vi "MoveMultiDrives.vi"(0 "Start Counter":dbl[](array[numeric]), 1 "Channel Properties":T1[](array[typedef]) {"Current Pos" format="%.2f"; "Backlash/Eng units" format="%.2f"; "Pulses/rev" format="%.2f"; "Pos Tolerance" format="%.2f"; "Pulses/unit" format="%.2f"; "Acc. Min" format="%.2f"; "Acc. Max" format="%.2f"; "Vel. Min" format="%.2f"; "Vel. Max" format="%.2f"; "Acc. Default" format="%.2f"; "Vel. Default" format="%.2f"}, 2 "GoTo Array (pulse position, some channels)":T4[](array[typedef]) {"Acceleration" format="%.2f"; "Velocity" format="%.2f"; "Go To Position" step=100000.0}, 3 "Final move":bool, 4 "Predicted Move Time":dbl format="%.2f") -> (5 "Error string":string, 6 "Stop Pressed?":bool, 7 "Channel Properties Out":T1[](array[typedef]) {"Current Pos" format="%.2f"; "Backlash/Eng units" format="%.2f"; "Pulses/rev" format="%.2f"; "Pos Tolerance" format="%.2f"; "Pulses/unit" format="%.2f"; "Acc. Min" format="%.2f"; "Acc. Max" format="%.2f"; "Vel. Min" format="%.2f"; "Vel. Max" format="%.2f"; "Acc. Default" format="%.2f"; "Vel. Default" format="%.2f"})   [LabVIEW 2022 SP3]
uses:
  ~subVIs/DriveClusterLower.ctl
  ~subVIs/DriveStatus.ctl
  ~subVIs/DriveProperties.ctl
  ~subVIs/Traverse Type.ctl
  ~subVIs/GenericDriveCommand.ctl
  Dynamixel/Sub Vis/Dynamixel Commands.ctl
  ~subVIs/DriveConfigGlobal.vi
  Anemometry/Anemometry Sub Vis/Globals/Trav_pos_global.vi
panel:
  out "Actual Travel Time":dbl format="%#.3g"
  out "Case":string
  out "Working?":bool
  out "ErrorMagnitude":dbl
  out "Move On Track?":bool
  out "Log File":path
  out "Move Terminated on Timeout":bool
  in  "Axis info cluster":T3
  out "Start Time":dbl format="%.2f"
  out "Bar2":dbl(slide)=2.0 scale=-23355.245670318604..-23317.840270996094
  out "Bar1":dbl(slide)=2.0 scale=-142950.39999389648..-143360.0
  out "Bar0":dbl(slide)=2.0 scale=228853.125..229365.0
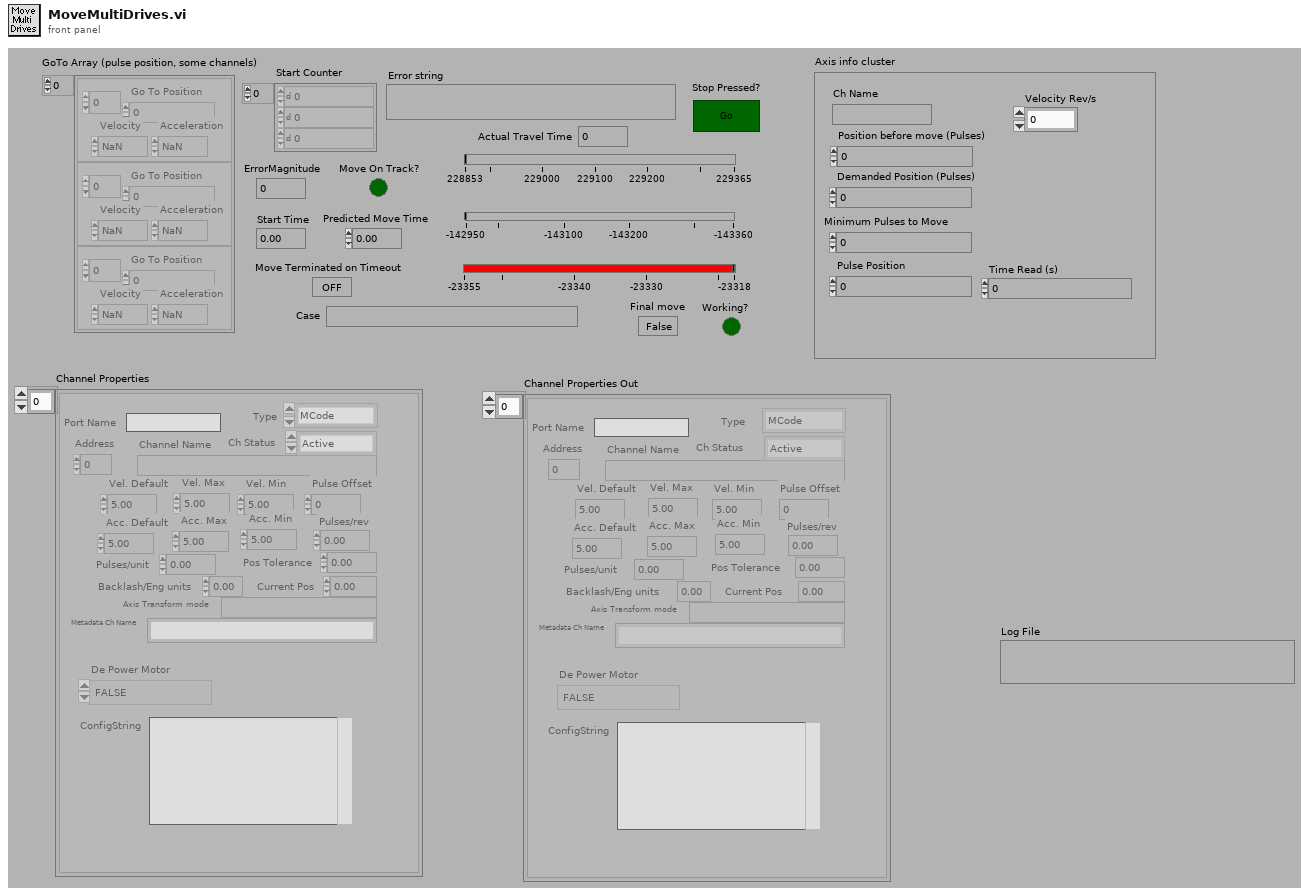
[diagram p1: front panel]
types:
  T1 = typedef "DriveProperties.ctl" = cluster{"Channel Name":string, "Vel. Default":sgl, "Acc. Default":sgl, "Vel. Max":sgl, "Vel. Min":sgl, "Acc. Max":sgl, "Acc. Min":sgl, "Pulses/unit":sgl, "Address":u8, "Pulse Offset":i32, "Pos Tolerance":sgl, "Pulses/rev":sgl, "Backlash/Eng units":sgl, "Current Pos":sgl, "Ch Status":enum16{"Active", "Offline", "Simulate"}, "Port Name":string, "Axis Transform mode":string, "Metadata Ch Name":string, "Type":T2, "De Power Motor":enum16{"TRUE", "FALSE"}, "ConfigString":string}
  T2 = typedef "Traverse Type.ctl" = enum16{"MCode", "Dynamixel"}
  T3 = typedef "DriveStatus.ctl" = cluster{"Ch Name":string, "Position before move (Pulses)":dbl, "Demanded Position (Pulses)":dbl, "Minimum Pulses to Move":dbl, "Pulse Position":dbl, "Time Read (s)":dbl, "Velocity Rev/s":dbl}
  T4 = typedef "DriveClusterLower.ctl" = cluster{"Go To Position":dbl, "Velocity":dbl, "Acceleration":dbl, "Address":u8}
  T5 = typedef "GenericDriveCommand.ctl" = string
  T6 = typedef "Dynamixel Commands.ctl" = enum16{"Torque Enable", "Present Position", "Threshold", "Max Position Limit", "Acceleration Profile", "Velocity Profile", "Goal Position", "Position Proportional Gain", "Position Integral Gain", "Position Differential Gain ", "Shutdown", "Write Operating Mode", "Read Operating Mode"}
  T7 = cluster{"GenericDriveCommand":T5, "Go To Position":dbl}
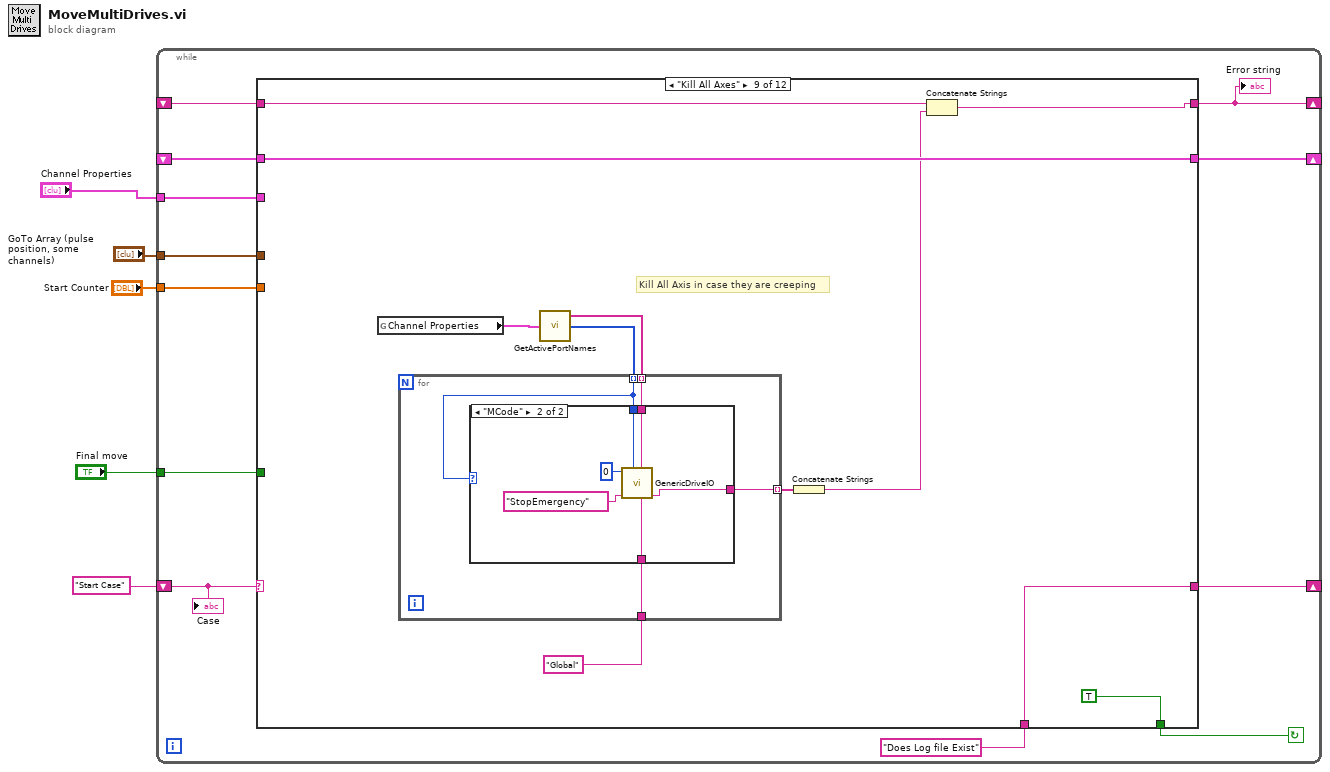
[diagram p0: block diagram]
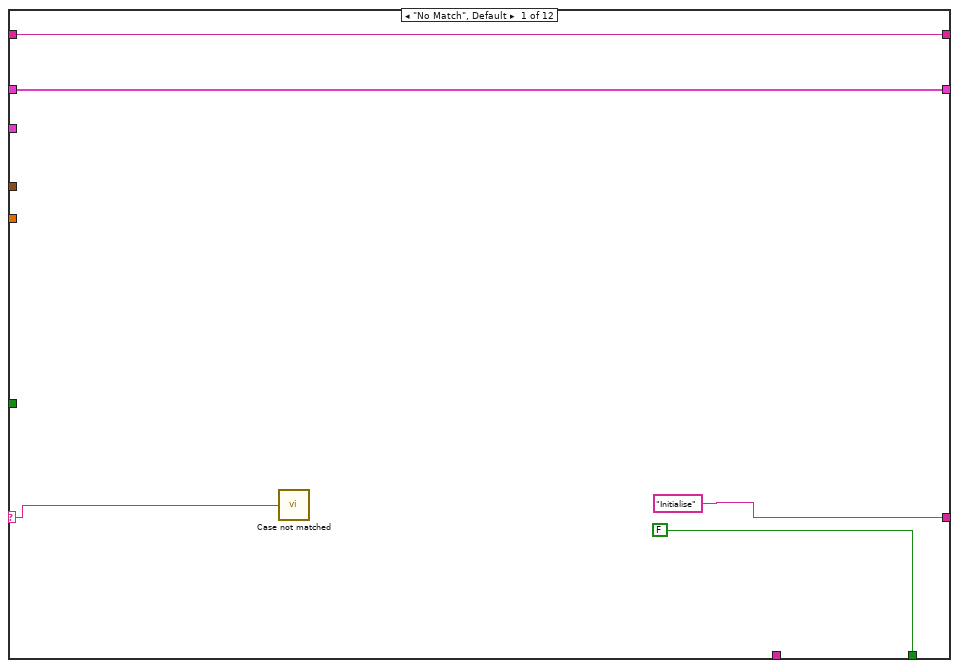
[diagram p2: hidden frame]
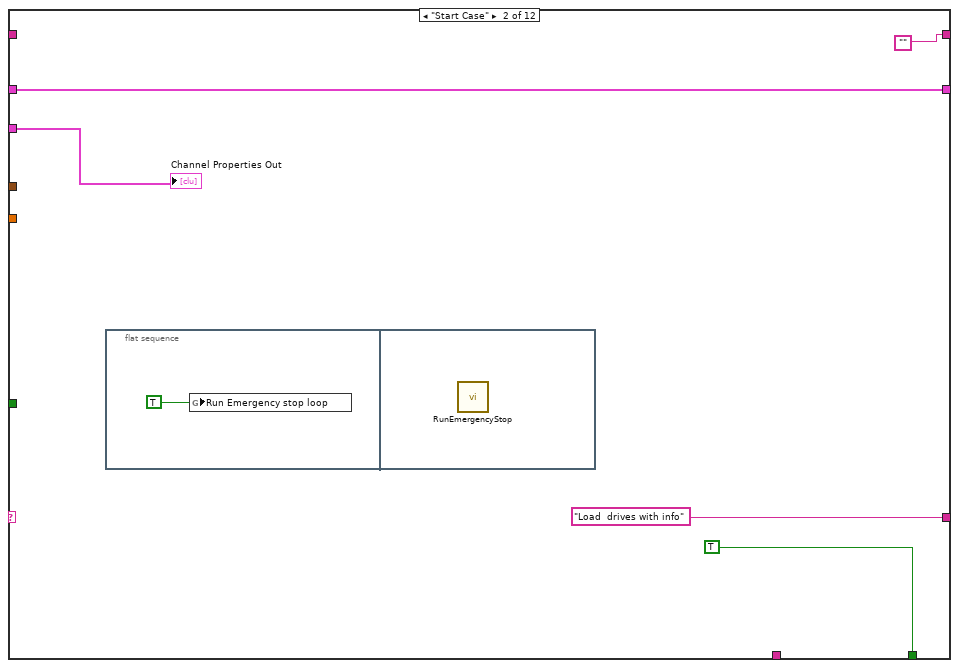
[diagram p3: hidden frame]
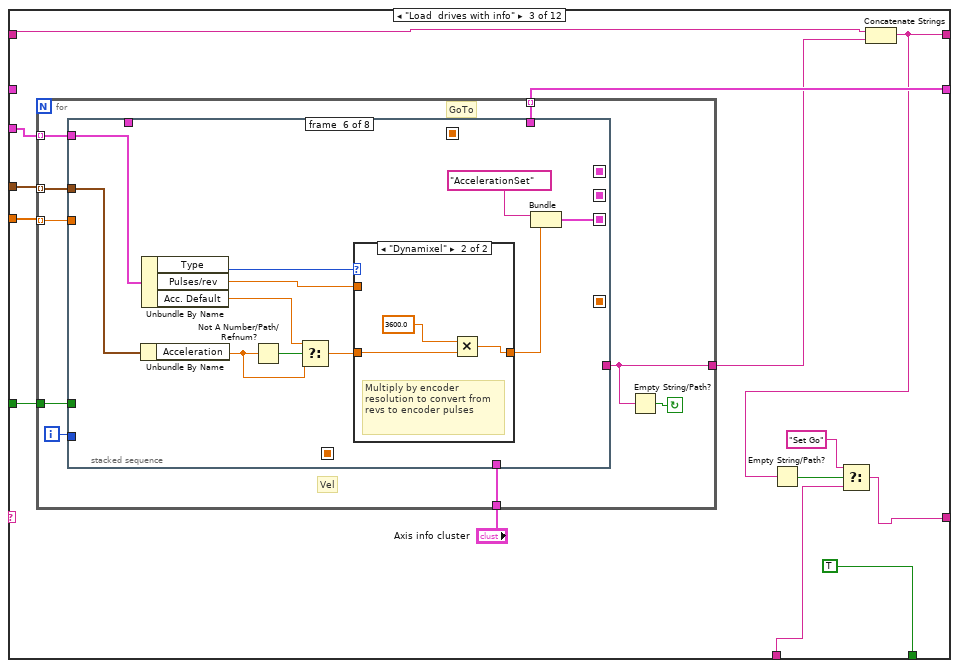
[diagram p4: hidden frame]
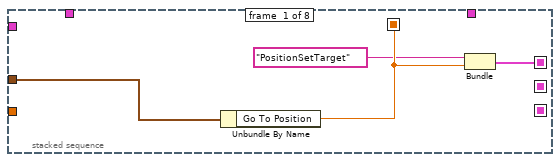
[diagram p5: hidden frame]
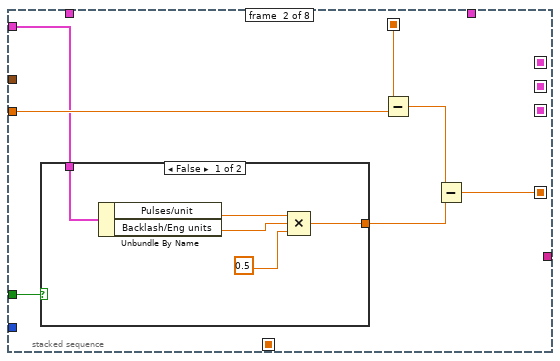
[diagram p6: hidden frame]
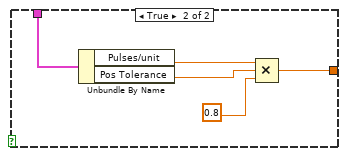
[diagram p7: hidden frame]
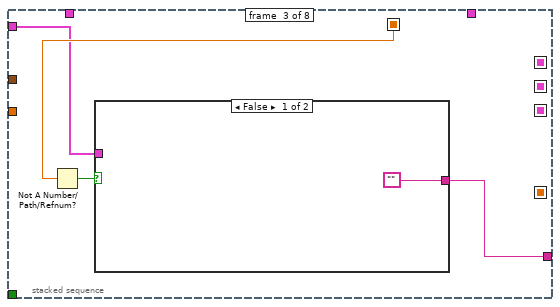
[diagram p8: hidden frame]
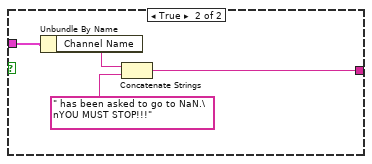
[diagram p9: hidden frame]
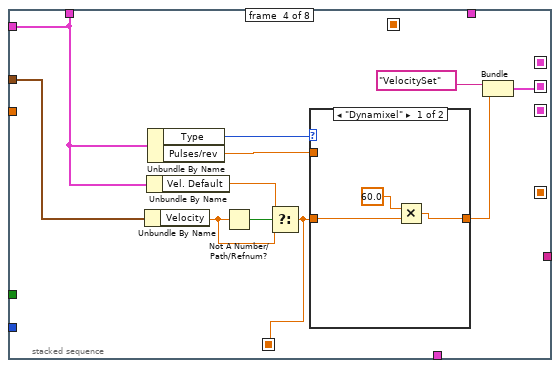
[diagram p10: hidden frame]
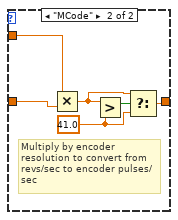
[diagram p11: hidden frame]
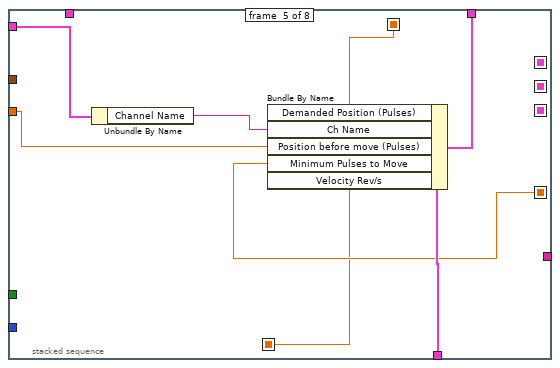
[diagram p12: hidden frame]
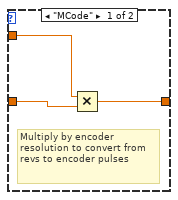
[diagram p13: hidden frame]
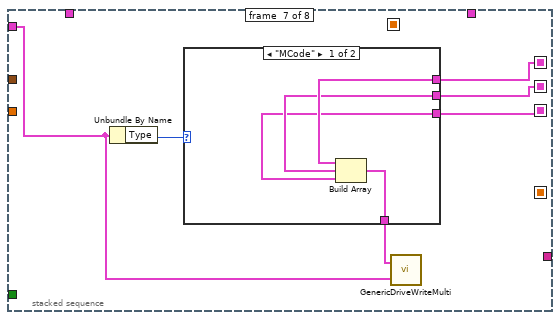
[diagram p14: hidden frame]
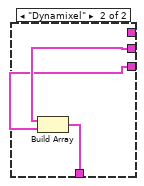
[diagram p15: hidden frame]
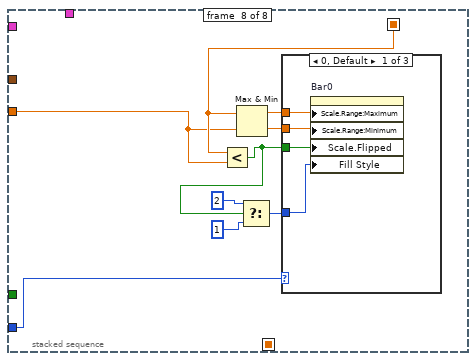
[diagram p16: hidden frame]
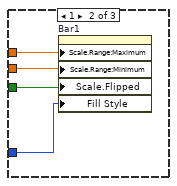
[diagram p17: hidden frame]
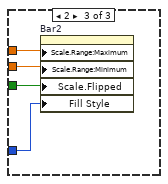
[diagram p18: hidden frame]
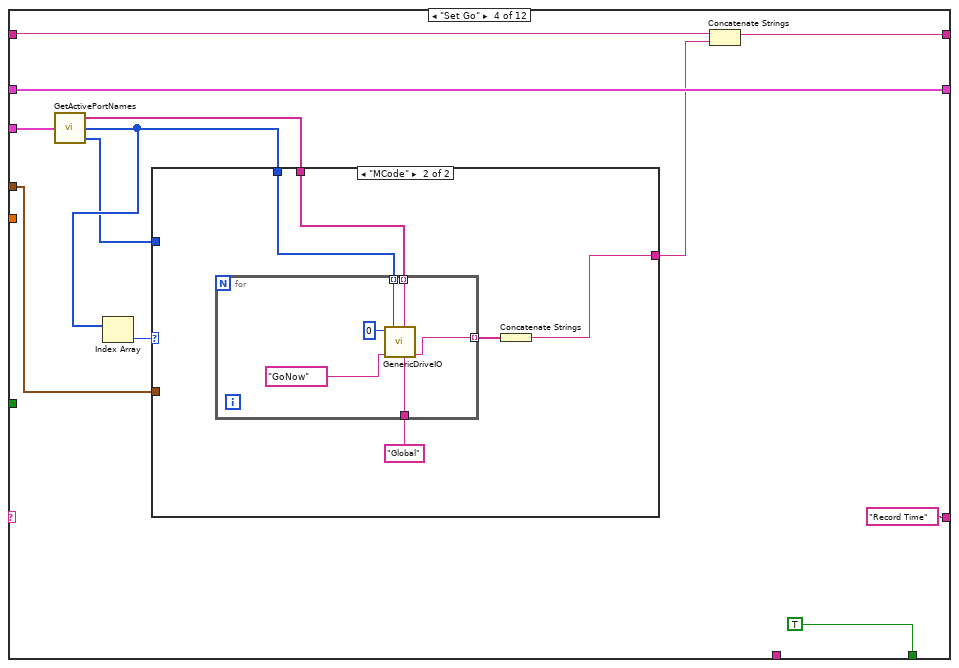
[diagram p19: hidden frame]
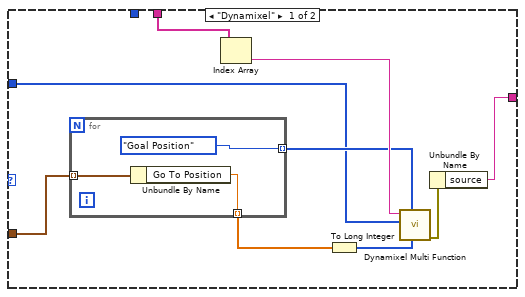
[diagram p20: hidden frame]
diagram:
  n1 = while {
    shift-left: _ -> [w12]
    shift-right: [w11] -> _
    tunnel: "Final move" -> [w13]
    tunnel: "Start Counter" -> [w14]
    tunnel: "GoTo Array (pulse position, some channels)" -> [w15]
    tunnel: "Channel Properties" -> [w16]
    shift-left: "Start Case" -> [w17]
    shift-right: [w7] -> _
    shift-right: [w6] -> _
    shift-left: _ -> [w10]
    stop <- w9 continue-if-true
    n2 = case shown="\"Kill All Axes\"" w17 {
      selector: w17 -> [w19 _ _ _ _ _ _ _ _ _ _ _]
      tunnel: [FALSE TRUE TRUE TRUE TRUE TRUE TRUE TRUE TRUE TRUE TRUE FALSE] -> w9
      tunnel: ["Initialise" "Load  drives with info" w30 "Record Time" "Check status of axis" w209 "Continue looping?" w359 w391 w419 "Write to Log file" "End"] -> w7
      tunnel: w16 -> [_ w23 w29 w162 _ w204 w253 w355 _ _ _ _]
      tunnel: w15 -> [_ _ w41 w163 _ _ w261 w353 _ _ _ _]
      tunnel: w14 -> [_ _ w40 _ _ _ w260 _ _ _ _ _]
      tunnel: w13 -> [_ _ w39 _ _ _ _ _ _ _ _ _]
      tunnel: [w20 w25 w37 w170 w199 w218 w259 w362 w395 w414 w441 w463] -> w11
      tunnel: w12 -> [w20 w25 _ w170 w199 w203 w259 w362 w395 w414 w441 w463]
      tunnel: w10 -> [w18 _ w36 w168 w197 w207 w256 w338 w389 w415 w423 w462]
      tunnel: [w18 "" w34 w167 w197 w205 w254 w338 w387 w415 w423 w462] -> w6
      tunnel: "Does Log file Exist" -> [_ _ w31 _ _ _ _ _ w391 _ _ _]
      frame "No Match", Default {
        n3 = call "Case not matched.vi"("Case Name not Matched"=w19) -> ()
      }
      frame "Start Case" {
        n4 = flat-sequence {
          frame #0 {
            n5 = global write "DriveConfigGlobal.vi" "Run Emergency stop loop"(TRUE) -> ()
          }
          frame #1 {
            n6 = call "RunEmergencyStop.vi"() -> ()  [unwired: 1 in, 7 out]
          }
        }
        "Channel Properties Out" <- w23
      }
      frame "Load  drives with info" {
        n7 = for {
          tunnel: w41 -> [w50] mode=indexing
          tunnel: w40 -> [w49] mode=indexing
          tunnel: w39 -> [w48]
          tunnel: "Axis info cluster" -> [w47]
          tunnel: [w46] -> w37 mode=indexing
          tunnel: [w45] -> w35
          tunnel: w29 -> [w43] mode=indexing
          i -> [w51]
          stop <- w44 continue-if-true
          # "Vel"
          # "GoTo"
          n8 = stacked-sequence {
            seq-local: [w54 _ _ _ _ _ _ _] -> [_ w62 w76 _ w104 _ _ w145]
            seq-local: [w53 _ _ _ _ _ _ _] -> [_ _ _ _ _ _ w132 _]
            seq-local: [_ _ _ w88 _ _ _ _] -> [_ _ _ _ _ _ w131 _]
            seq-local: [_ _ _ _ _ w117 _ _] -> [_ _ _ _ _ _ w130 _]
            seq-local: [_ w58 _ _ _ _ _ _] -> [_ _ _ _ w108 _ _ _]
            seq-local: [_ _ _ w83 _ _ _ _] -> [_ _ _ _ w103 _ _ _]
            tunnel: w50 -> [w55 _ _ w92 _ w120 _ _]
            tunnel: w51 -> [_ _ _ _ _ _ _ w146]
            tunnel: w48 -> [_ w60 _ _ _ _ _ _]
            tunnel: [_ _ _ w82 _ _ _ _] -> _
            tunnel: w49 -> [_ w59 _ _ w106 _ _ w144]
            tunnel: w47 -> [_ _ _ _ w109 _ _ _]
            tunnel: [_ _ _ _ w107 _ _ _] -> w46
            tunnel: [_ _ w74 _ _ _ _ _] -> w45
            tunnel: w43 -> [_ w56 w73 w82 w102 w112 w127 _]
            frame #0 {
              n9 = Unbundle By Name(w55) -> ("Go To Position"=w54:dbl)
              n10 = Bundle("GenericDriveCommand"=T5 "PositionSetTarget", "Go To Position"=w54) -> (w53:T7)  [unwired: 1 out]
            }
            frame #1 {
              n11 = case shown="False" w60 {
                tunnel: w56 -> [w67 w72]
                tunnel: [w63 w68] -> w61
                frame False {
                  n12 = Unbundle By Name(w67) -> ("Pulses/unit"=w66:sgl, "Backlash/Eng units"=w65:sgl)
                  n13 = Compound Arithmetic op=MULTIPLY(w66, w65, 0.5) -> (w63:dbl)
                }
                frame True {
                  n14 = Unbundle By Name(w72) -> ("Pulses/unit"=w71:sgl, "Pos Tolerance"=w70:sgl)
                  n15 = Compound Arithmetic op=MULTIPLY(w71, w70, 0.8) -> (w68:dbl)
                }
              }
              n16 = Subtract(x=w62, y=w59) -> (x-y=w57:dbl)
              n17 = Subtract(x=w57, y=w61) -> (x-y=w58:dbl)
            }
            frame #2 {
              n18 = Not A Number/Path/Refnum?(number/path/refnum=w76) -> (NaN/Path/Refnum?=w75:bool)
              n19 = case shown="False" w75 {
                tunnel: w73 -> [_ w81]
                tunnel: ["" w80] -> w74
                frame False {
                }
                frame True {
                  n20 = Unbundle By Name(w81) -> ("Channel Name"=w79:string)
                  n21 = Concatenate Strings(w79, " has been asked to go to NaN.\nYOU MUST STOP!!!") -> (w80:string)
                }
              }
            }
            frame #3 {
              n22 = Unbundle By Name(w92) -> ("Velocity"=w89:dbl)
              n23 = Unbundle By Name(w82) -> ("Vel. Default"=w90:sgl)
              n24 = Unbundle By Name(w82) -> ("Type"=w86:T2, "Pulses/rev"=w85:sgl)
              n25 = Not A Number/Path/Refnum?(number/path/refnum=w89) -> (NaN/Path/Refnum?=w91:bool)
              n26 = Select(t=w90, s=w91, f=w89) -> (s? t:f=w83:dbl)
              n27 = case shown="\"Dynamixel\"" w86 {
                tunnel: w83 -> [w95 w96]
                tunnel: w85 -> [_ w101]
                tunnel: [w93 w100] -> w84
                frame "Dynamixel" {
                  n28 = Multiply(x=60.0, y=w95) -> (x*y=w93:dbl)
                }
                frame "MCode" {
                  w97 = 41.0 ("y")
                  # "Multiply by encoder resolution to convert from revs/sec to encoder pulses/sec"
                  n29 = Multiply(x=w101, y=w96) -> (x*y=w98:dbl)
                  n30 = Greater?(x=w98, y=w97) -> (0:w99:bool)
                  n31 = Select(t=w98, s=w99, f=w97) -> (s? t:f=w100:dbl)
                }
              }
              n32 = Bundle("GenericDriveCommand"=T5 "VelocitySet", "y"=w84) -> (w88:cluster{"GenericDriveCommand":T5, "y":dbl})  [unwired: 1 out]
            }
            frame #4 {
              n33 = Unbundle By Name(w102) -> ("Channel Name"=w105:string)
              n34 = Bundle By Name(cluster=w109, "Demanded Position (Pulses)"=w104, "Ch Name"=w105, "Position before move (Pulses)"=w106, "Minimum Pulses to Move"=w108, "Velocity Rev/s"=w103) -> (w107:T3)
            }
            frame #5 {
              n35 = Unbundle By Name(w120) -> ("Acceleration"=w118:dbl)
              n36 = Unbundle By Name(w112) -> ("Type"=w111:T2, "Pulses/rev"=w115:sgl, "Acc. Default"=w110:sgl)
              n37 = Not A Number/Path/Refnum?(number/path/refnum=w118) -> (NaN/Path/Refnum?=w119:bool)
              n38 = Select(t=w110, s=w119, f=w118) -> (s? t:f=w114:dbl)
              n39 = case shown="\"Dynamixel\"" w111 {
                tunnel: w114 -> [w123 w126]
                tunnel: w115 -> [w121 _]
                tunnel: [w122 w124] -> w113
                frame "MCode" {
                  # "Multiply by encoder resolution to convert from revs to encoder pulses"
                  n40 = Multiply(x=w121, y=w123) -> (x*y=w122:dbl)
                }
                frame "Dynamixel" {
                  # "Multiply by encoder resolution to convert from revs to encoder pulses"
                  n41 = Multiply(x=3600.0, y=w126) -> (x*y=w124:dbl)
                }
              }
              n42 = Bundle("GenericDriveCommand"=T5 "AccelerationSet", w113) -> (w117:cluster{"GenericDriveCommand":T5, dbl})  [unwired: 1 out]
            }
            frame #6 {
              n43 = Unbundle By Name(w127) -> ("Type"=w128:T2)
              n44 = case shown="\"MCode\"" w128 {
                tunnel: w132 -> [w136 _]
                tunnel: w131 -> [w135 w139]
                tunnel: w130 -> [w134 w138]
                tunnel: [w133 w137] -> w129
                frame "MCode" {
                  n45 = Build Array(w136, w135, w134) -> (w133:cluster{"GenericDriveCommand":T5, "y":dbl}[])
                }
                frame "Dynamixel" {
                  n46 = Build Array(w139, w138) -> (w137:cluster{"GenericDriveCommand":T5, "y":dbl}[])
                }
              }
              n47 = call "GenericDriveWriteMulti.vi"("Channel Description"=w127, "Array Constant"=w129) -> ()  [unwired: 4 in, 1 out]
            }
            frame #7 {
              n48 = Less?(x=w145, y=w144) -> (x < y?=w143:bool)
              n49 = Max & Min(x=w145, y=w144) -> (max(x,y)=w148:dbl, min(x,y)=w147:dbl)
              n50 = Select(t=2, s=w143, f=1 ("Fill Style")) -> (s? t:f=w140:i32)
              n51 = case shown="0, Default" w146 {
                tunnel: w148 -> [w152 w156 w160]
                tunnel: w147 -> [w151 w155 w159]
                tunnel: w143 -> [w150 w154 w158]
                tunnel: w140 -> [w149 w153 w157]
                frame 0, Default {
                  n52 = property on="Bar0" class="Slide (strict)"("Scale.Range:Maximum"=w152, "Scale.Range:Minimum"=w151, "Scale.Flipped"=w150, "Fill Style"=w149) -> ()  [unwired: 2 in, 2 out]
                }
                frame 1 {
                  n53 = property on="Bar1" class="Slide (strict)"("Scale.Range:Maximum"=w156, "Scale.Range:Minimum"=w155, "Scale.Flipped"=w154, "Fill Style"=w153) -> ()  [unwired: 2 in, 2 out]
                }
                frame 2 {
                  n54 = property on="Bar2" class="Slide (strict)"("Scale.Range:Maximum"=w160, "Scale.Range:Minimum"=w159, "Scale.Flipped"=w158, "Fill Style"=w157) -> ()  [unwired: 2 in, 2 out]
                }
              }
            }
          }
          n55 = Empty String/Path?(string/path=w45) -> (empty?=w44:bool)
        }
        n56 = Concatenate Strings(w36, w35) -> (w34:string)
        n57 = Empty String/Path?(string/path=w34) -> (empty?=w33:bool)
        n58 = Select(t="Set Go", s=w33, f=w31) -> (s? t:f=w30:string)
      }
      frame "Set Go" {
        n59 = call "GetActivePortNames.vi"("Channel Properties"=w162) -> ("Port Name Array"=w169:string[], "Drive Type Array"=w165:T2[], "Address"=w161:u8[])
        n60 = Index Array(array=w165) -> (element=w164:T2)  [unwired: 1 in]
        n61 = case shown="\"MCode\"" w164 {
          tunnel: w169 -> [w181 w188]
          tunnel: w165 -> [_ w187]
          tunnel: [w178 w185] -> w166
          tunnel: w163 -> [w177 _]
          tunnel: w161 -> [w173 _]
          frame "Dynamixel" {
            n62 = for {
              tunnel: w177 -> [w184] mode=indexing
              tunnel: [Dynamixel_Commands."Goal Position" ("Function")] -> w176 mode=indexing
              tunnel: [w182] -> w175 mode=indexing
              n63 = Unbundle By Name(w184) -> ("Go To Position"=w182:dbl)
            }
            n64 = Index Array(array=w181) -> (element=w180:string)  [unwired: 1 in]
            n65 = To Long Integer(number=w175) -> (32bit integer=w174:i32[])
            n66 = call "Dynamixel Multi Function.vi"("Data Array"=w174, "Function Array"=w176, "Motor ID"=w173, "Com port"=w180) -> ("error out"=w179:errorcluster)  [unwired: 6 in, 1 out]
            n67 = Unbundle By Name(w179) -> ("source"=w178:string)
          }
          frame "MCode" {
            n68 = for {
              tunnel: w188 -> [w195] mode=indexing
              tunnel: "Global" -> [w194]
              tunnel: w187 -> [w193] mode=indexing
              tunnel: [w191] -> w186 mode=indexing
              n69 = call "GenericDriveIO.vi"("GenericDriveCommand"=T5 "GoNow", "Channel Name"=w194, "Address"=u8 0, "Type"=w193, "Port Name"=w195) -> ("Error Description"=w191:string)  [unwired: 1 in, 5 out]
            }
            n70 = Concatenate Strings(w186) -> (w185:string)
          }
        }
        n71 = Concatenate Strings(w168, w166) -> (w167:string)
      }
      frame "Record Time" {
        n72 = Get Date/Time In Seconds() -> (seconds since 1Jan1904=w198:timestamp)
        n73 = To Double Precision Float(number=w198) -> (double precision float=→"Start Time":dbl)
        n74 = Wait (ms)(milliseconds to wait=u32 50) -> ()  [unwired: 1 out]
      }
      frame "Check status of axis" {
        (unwired) "Global"
        n75 = global read "Trav_pos_global.vi" "Live Channel Position"() -> (w215:sgl[])
        n76 = for {
          shift-right: [w239] -> w206
          shift-left: "" -> [w240]
          tunnel: w204 -> [w220] mode=indexing
          tunnel: [w238] -> w218 mode=indexing
          shift-right: [w236] -> w213
          shift-left: w215 -> [w237]
          tunnel: [w222] -> w212
          tunnel: w203 -> [w221] mode=indexing
          i -> [w241]
          n77 = Unbundle By Name(w220) -> ("Channel Name"=w231:string, "Pulses/unit"=w234:sgl, "Pulse Offset"=w232:i32)
          n78 = call "CheckDriveStatus.vi"("Channel Properties"=w220, "Axis info cluster"=w221) -> ("Error string"=w235:string, "Axis info cluster Out"=w238:T3)
          n79 = Unbundle By Name(w238) -> ("Pulse Position"=w226:dbl)
          n80 = Match Pattern(string=w231, regular expression=":") -> (before substring=w222:string, after substring=w228:string)  [unwired: 1 in, 2 out]
          n81 = Match Pattern(string=w228, regular expression=":") -> (after substring=w227:string)  [unwired: 1 in, 3 out]
          n82 = Add(x=w232, y=w226) -> (x+y=w233:dbl)
          n83 = case shown="\"Z\", Default" w227 {
            tunnel: [0 1 2] -> w225
            frame "X" {
            }
            frame "Y" {
            }
            frame "Z", Default {
            }
          }
          n84 = Divide(x=w233, y=w234) -> (x/y=w224:dbl)
          n85 = Not A Number/Path/Refnum?(number/path/refnum=w224) -> (NaN/Path/Refnum?=w223:bool)
          n86 = case shown="False" w223 {
            tunnel: w237 -> [w245 w246]
            tunnel: w224 -> [w244 _]
            tunnel: w225 -> [w243 _]
            tunnel: [w242 w246] -> w236
            frame False {
              n87 = Replace Array Subset(array=w245, new element=w244, index=w243) -> (w242:sgl[])
            }
            frame True {
            }
          }
          n88 = Concatenate Strings(w240, w235) -> (w239:string)
          n89 = case shown="2" w241 {
            tunnel: w226 -> [w250 w251 w252]
            frame 0, Default {
              "Bar0" <- w250
            }
            frame 1 {
              "Bar1" <- w251
            }
            frame 2 {
              "Bar2" <- w252
            }
          }
        }
        n90 = global write "Trav_pos_global.vi" "Live Channel Position"(w213) -> ()
        n91 = call "Coordinate_transforms.vi"("Traverse Name"=w212, "Input"=w213, "Mode"=enum16{"XYZ to Channel", "Channel to XYZ"}."Channel to XYZ") -> ("Output"=w214:sgl[])
        n92 = Empty String/Path?(string/path=w206) -> (empty?=w211:bool)
        n93 = global write "Trav_pos_global.vi" "Live Position"(w214) -> ()
        n94 = Concatenate Strings(w207, w206) -> (w205:string)
        n95 = Select(t="Is Move On track?", s=w211, f="Continue looping?") -> (s? t:f=w209:string)
      }
      frame "Is Move On track?" {
        n96 = stacked-sequence {
          seq-local: [w262 _ _] -> [_ w277 _]
          seq-local: [_ w273 _] -> [_ _ w333]
          tunnel: w261 -> [w266 w274 _]
          tunnel: w260 -> [w265 w276 _]
          tunnel: w259 -> [_ w275 _]
          tunnel: [_ _ w332] -> w255
          tunnel: w253 -> [_ w272 _]
          frame #0 {
            n97 = for {
              tunnel: w266 -> [w271] mode=indexing
              tunnel: w265 -> [w269] mode=indexing
              tunnel: [w267] -> w264 mode=indexing
              n98 = Unbundle By Name(w271) -> ("Go To Position"=w270:dbl)
              n99 = Subtract(x=w270, y=w269) -> (x-y=w268:dbl)
              n100 = Absolute Value(x=w268) -> (abs(x)=w267:dbl)
            }
            n101 = call "Sort_Array_Indicies.vi"("unsorted array"=w264) -> ("Sort Index"=w263:i32[])  [unwired: 1 out]
            n102 = Reverse 1D Array(array=w263) -> (reversed array=w262:i32[])
          }
          frame #1 {
            n103 = for {
              shift-right: [w297] -> _
              shift-left: _ -> [w298]
              tunnel: [w294] -> w273
              tunnel: w272 -> [w293]
              tunnel: w277 -> [w285] mode=indexing
              tunnel: w276 -> [w290]
              tunnel: w275 -> [w289]
              tunnel: w274 -> [w288]
              shift-right: [w281] -> _
              shift-left: _ -> [w279]
              i -> [w299]
              # "Would be nice to make this truly a mm deviation from straight?"
              n104 = Index Array(array=w289, index=w285) -> (element=w286:T3)
              n105 = Index Array(array=w288, index=w285) -> (element=w287:T4)
              n106 = Index Array(array=w290, index=w285) -> (element=w291:dbl)
              n107 = Index Array(array=w293, index=w285) -> (element=w292:T1)
              n108 = Unbundle By Name(w287) -> ("Go To Position"=w302:dbl)
              n109 = Unbundle By Name(w286) -> ("Velocity Rev/s"=w278:dbl, "Ch Name"=w283:string, "Pulse Position"=w301:dbl, "Time Read (s)"=w280:dbl)
              n110 = Subtract(x=w302, y=w291) -> (x-y=w295:dbl)
              n111 = Subtract(x=w301, y=w291) -> (x-y=w300:dbl)
              n112 = Match Pattern(string=w283, regular expression=":") -> (before substring=w282:string)  [unwired: 1 in, 3 out]
              n113 = Divide(x=w300, y=w295) -> (x/y=w296:dbl)
              n114 = case shown="1, Default" w299 {
                tunnel: [w305 w328] -> w297
                tunnel: w298 -> [_ w328]
                tunnel: w296 -> [w305 w331]
                tunnel: w295 -> [_ w329]
                tunnel: [TRUE w325] -> w294
                tunnel: w292 -> [_ w322]
                tunnel: w282 -> [_ w318]
                tunnel: [w303 w316] -> w281
                tunnel: w280 -> [w303 w317]
                tunnel: w279 -> [_ w316]
                tunnel: w278 -> [_ w315]
                frame 0 {
                }
                frame 1, Default {
                  # "Error in mm"
                  # "Error in Revs"
                  # "Loads tolerance from file"
                  n115 = Subtract(x=w331, y=w328) -> (x-y=w330:dbl)
                  n116 = Unbundle By Name(w322) -> ("Pulses/unit"=w311:sgl, "Pulses/rev"=w313:sgl)
                  n117 = Subtract(x=w317, y=w316) -> (x-y=w308:dbl)
                  n118 = Multiply(x=w329, y=w330) -> (x*y=w323:dbl)
                  n119 = Multiply(x=w315, y=w308) -> (x*y=w314:dbl)
                  n120 = Divide(x=w323, y=w311) -> (x/y=w321:dbl)
                  n121 = call "SetMoveTolerance.vi"("Traverse Name"=w318) -> ("Max Error in Eng Units"=w319:u32)
                  n122 = Absolute Value(x=w321) -> (abs(x)=w320:dbl)
                  "ErrorMagnitude" <- w320
                  n123 = To Double Precision Float(number=w319) -> (double precision float=w310:dbl)
                  n124 = Multiply(x=w313, y=w314) -> (x*y=w312:dbl)
                  n125 = Divide(x=w312, y=w311) -> (x/y=w307:dbl)
                  n126 = Not A Number/Path/Refnum?(number/path/refnum=w320) -> (NaN/Path/Refnum?=w327:bool)
                  n127 = Absolute Value(x=w307) -> (abs(x)=w306:dbl)
                  n128 = Add(x=w310, y=w306) -> (x+y=w309:dbl)
                  n129 = Less?(x=w320, y=w309) -> (x < y?=w326:bool)
                  n130 = Select(t=TRUE, s=w327, f=w326) -> (s? t:f=w325:bool)
                }
              }
            }
            "Move On Track?" <- w273
          }
          frame #2 {
            n131 = case shown="False" w333 {
              tunnel: ["Move Stopped due to axes not being in the correct positions relative to one another during move" ""] -> w332
              frame False {
              }
              frame True {
              }
            }
          }
        }
        n132 = Concatenate Strings(w256, w255) -> (w254:string)
      }
      frame "Continue looping?" {
        n133 = for {
          tunnel: w362 -> [w385] mode=indexing
          tunnel: [w380] -> w350 mode=indexing
          tunnel: w355 -> [w384] mode=indexing
          tunnel: w353 -> [w383] mode=indexing
          tunnel: [w377] -> w352 mode=indexing
          n134 = Unbundle By Name(w383) -> ("Go To Position"=w379:dbl)
          n135 = Unbundle By Name(w385) -> ("Pulse Position"=w380:dbl)
          n136 = Unbundle By Name(w384) -> ("Pulses/unit"=w382:sgl, "Pos Tolerance"=w381:sgl)
          n137 = Multiply(x=w382, y=w381) -> (x*y=w378:sgl)
          n138 = Add(x=w379, y=w378) -> (x+y=w376:dbl)
          n139 = Subtract(x=w379, y=w378) -> (x-y=w375:dbl)
          n140 = Build Array(w376, w375) -> (w374:dbl[])
          n141 = Array Max & Min(array=w374) -> (max value=w373:dbl, min value=w372:dbl)  [unwired: 2 out]
          n142 = In Range and Coerce(upper limit=w373, x=w380, lower limit=w372) -> (In Range?=w377:bool)  [unwired: 1 out]
        }
        n143 = Multiply(x="Predicted Move Time", y=1.1) -> (x*y=w367:dbl)
        n144 = Add(x=w367, y=10.0) -> (x+y=w364:dbl)
        n145 = local read "Start Time"() -> (w363:dbl)
        n146 = Get Date/Time In Seconds() -> (seconds since 1Jan1904=w356:timestamp)
        n147 = To Double Precision Float(number=w356) -> (double precision float=w345:dbl)
        n148 = Subtract(x=w345, y=w363) -> (x-y=w344:dbl)
        "Actual Travel Time" <- w344
        n149 = call "Program_Active.vi"() -> ()  [unwired: 1 in]
        n150 = Multiply(x="Predicted Move Time", y=0.7) -> (x*y=w343:dbl)
        n151 = Match Pattern(string=w338, regular expression="Motion stopped") -> (offset past match=w337:i32)  [unwired: 1 in, 3 out]
        n152 = Less?(x=w344, y=w364) -> (x < y?=w358:bool)
        n153 = Greater?(x=w344, y=w343) -> (0:w342:bool)
        n154 = Greater Or Equal To 0?(x=w337) -> (x >= 0?=w336:bool)
        n155 = Not(x=w358) -> (.not. x?=→"Move Terminated on Timeout":bool)
        n156 = And Array Elements(Boolean array=w352) -> (logical AND=w348:bool)
        n157 = while {
          shift-right: [w371] -> _
          shift-left: _ -> [_]
          shift-left: _ -> [w369]
          tunnel: w350 -> [w371]
          tunnel: [w369] -> w349
          stop <- TRUE stop-if-true
        }
        n158 = Equal?(x=w349, y=w350) -> (x = y?=w341:bool)
        n159 = And(x=w341, y=w342) -> (x .and. y?=w340:bool)
        n160 = global read "DriveConfigGlobal.vi" "Stop Pressed?"() -> (w354:bool)
        "Stop Pressed?" <- w354
        n161 = Compound Arithmetic op=AND(invert w336, invert w354, invert w340, invert w348, w358) -> (w351:bool)
        "Working?" <- w351
        n162 = Select(t="Check status of axis", s=w351, f="Kill All Axes") -> (s? t:f=w359:string)
      }
      frame "Kill All Axes" {
        # "Kill All Axis in case they are creeping"
        n163 = global read "DriveConfigGlobal.vi" "Channel Properties"() -> (w386:T1[])
        n164 = call "GetActivePortNames.vi"("Channel Properties"=w386) -> ("Port Name Array"=w394:string[], "Drive Type Array"=w392:T2[])  [unwired: 1 out]
        n165 = for {
          tunnel: w394 -> [w400] mode=indexing
          tunnel: "Global" -> [w399]
          tunnel: w392 -> [w397] mode=indexing
          tunnel: [w398] -> w390 mode=indexing
          n166 = case shown="\"MCode\"" w397 {
            tunnel: w400 -> [_ w407]
            tunnel: w399 -> [_ w406]
            tunnel: w397 -> [_ w405]
            tunnel: ["" w403] -> w398
            frame "Dynamixel" {
            }
            frame "MCode" {
              n167 = call "GenericDriveIO.vi"("GenericDriveCommand"=T5 "StopEmergency", "Channel Name"=w406, "Address"=u8 0, "Type"=w405, "Port Name"=w407) -> ("Error Description"=w403:string)  [unwired: 1 in, 5 out]
            }
          }
        }
        n168 = Concatenate Strings(w390) -> (w388:string)
        n169 = Concatenate Strings(w389, w388) -> (w387:string)
      }
      frame "Does Log file Exist" {
        n170 = Index Array(array=w414) -> (element=w413:T3)  [unwired: 1 in]
        n171 = Unbundle By Name(w413) -> ("Ch Name"=w412:string)
        n172 = Match Pattern(string=w412, regular expression=":") -> (before substring=w410:string)  [unwired: 1 in, 3 out]
        n173 = Concatenate Strings(w410, "_Low" ("Input Element")) -> (w408:string)
        n174 = call "Create_Error_log_folders.vi"("Log Filename"=w408, "Per Day Log File?"=TRUE) -> ("Local Log File"=→"Log File":path, "exists?"=w417:bool)  [unwired: 4 in]
        n175 = Select(t="Write to Log file", s=w417, f="Create Log file") -> (s? t:f=w419:string)
      }
      frame "Create Log file" {
        n176 = Build Array("Date::", "Time::", "Seconds:Since:1st Jan 1904", "Move:Duration:Seconds", "Move:Terminated:On Timeout") -> (w432:string[])
        n177 = for {
          N: 3 -> [_]
          shift-right: [w443] -> w431
          shift-left: w432 -> [w444]
          i -> [w449]
          n178 = Increment(x=w449) -> (x+1=w448:i32)
          n179 = Number To Decimal String(number=w448) -> (decimal integer string=w447:string)  [unwired: 1 out]
          n180 = Build Array("Axis:Ch Name:", "Position Before:Move (Pulses):", "Demanded:Position (Pulses):", "Minimum Pulses:to Move:", "Pulses:Moved:") -> (w446:string[])
          n181 = for {
            tunnel: w447 -> [w457]
            tunnel: w446 -> [w456] mode=indexing
            tunnel: [w455] -> w445 mode=indexing
            n182 = Concatenate Strings(w456, w457) -> (w455:string)
          }
          n183 = Build Array (concatenate)(w444, w445) -> (w443:string[])
        }
        n184 = for {
          tunnel: w431 -> [w461] mode=indexing
          tunnel: [w460] -> w435 mode=indexing
          tunnel: [w459] -> w436 mode=indexing
          tunnel: [w458] -> w437 mode=indexing
          n185 = call "Split_Ch_name.vi"("Ch name"=w461) -> ("Top level"=w460:string, "Middle"=w459:string, "Low level"=w458:string)
        }
        n186 = local read "Log File"() -> (w424:path)
        n187 = Build Array(w435, w436, w437) -> (w433:string[][])
        n188 = Array To Spreadsheet String(array=w433, 3:"%s" ("format string")) -> (spreadsheet string=w425:string)  [unwired: 1 out]
        n189 = call "Write_File_Simple.vi"("append to file? (new file:F)"=TRUE, "character string"=w425, "file path"=w424) -> ()  [unwired: 2 out]
      }
      frame "Write to Log file" {
        n190 = stacked-sequence {
          seq-local: [w470 _ _] -> [_ w482 _]
          seq-local: [_ w481 _] -> [_ _ w497]
          tunnel: w463 -> [_ w483 _]
          frame #0 {
            n191 = local read "Move Terminated on Timeout"() -> (w477:bool)
            n192 = Get Date/Time In Seconds() -> (seconds since 1Jan1904=w469:timestamp)
            n193 = local read "Start Time"() -> (w479:dbl)
            n194 = To Double Precision Float(number=w469) -> (double precision float=w468:dbl)
            n195 = Subtract(x=w468, y=w479) -> (x-y=w478:dbl)
            n196 = Get Date/Time String(date format (0)=enum16{"short", "long", "abbreviated"}."abbreviated", seconds (now)=w469) -> (date string=w474:string, time string=w473:string)  [unwired: 1 out]
            n197 = Number To Fractional String(number=w468, precision (6)=i16 3) -> (F-format string=w466:string)  [unwired: 2 out]
            n198 = Number To Decimal String(number=w478) -> (decimal integer string=w472:string)  [unwired: 1 out]
            n199 = Select(t="TRUE", s=w477, f="FALSE") -> (s? t:f=w471:string)
            n200 = Build Array(w474, w473, w466, w472, w471) -> (w470:string[])
          }
          frame #1 {
            n201 = for {
              tunnel: w483 -> [w493] mode=indexing
              shift-right: [w485] -> w481
              shift-left: w482 -> [w486]
              n202 = Unbundle By Name(w493) -> ("Ch Name"=w488:string, "Position before move (Pulses)"=w492:dbl, "Demanded Position (Pulses)"=w491:dbl, "Minimum Pulses to Move"=w484:dbl, "Pulse Position"=w490:dbl)
              n203 = Build Array(w492, w491, w484, w490) -> (w489:dbl[])
              n204 = Number To Decimal String(number=w489) -> (decimal integer string=w487:string[])  [unwired: 1 out]
              n205 = Build Array (concatenate)(w486, w488, w487) -> (w485:string[])
            }
          }
          frame #2 {
            n206 = for {
              shift-right: [w501] -> w494
              shift-left: "\r\n" -> [w502]
              tunnel: w497 -> [w500] mode=indexing
              n207 = Concatenate Strings(w502, w500, "\t") -> (w501:string)
            }
            n208 = local read "Log File"() -> (w495:path)
            n209 = call "Write_File_Simple.vi"("append to file? (new file:F)"=TRUE, "character string"=w494, "file path"=w495) -> ()  [unwired: 2 out]
          }
        }
      }
    }
    "Error string" <- w6
    "Case" <- w17
  }
